vi "BASE_I_O_Manual.vi"(8 "error in (no error)":errorcluster) -> (0 "error out":errorcluster)   [LabVIEW 2017]
doc: "This vi is for manually turn ON and OFF also monitor Output of PLCS. So this is manual screen."
uses:
  Global/PLC_to_Auto.vi
panel:
  in  "Tab Control":enum32{"MANUAL SWITCH", "SCANNER"}(tab)
  in  "Cluster - Thin Border":T1
  in  "Back":bool
  out "Input Signal":T2
  in  "Flush Scaner":bool
  out "SCANNED STRING":string
  in  "Leght of byte to read":bool
  in  "scan":bool
  out "SCANNED COM PORT":refnum<visa-resource-name>
  out "error out 3":errorcluster
  out "error out 4":errorcluster
  # "BARCODE VERIFICATION SYSTEM REPORTS"
  # "Manual Cycle"
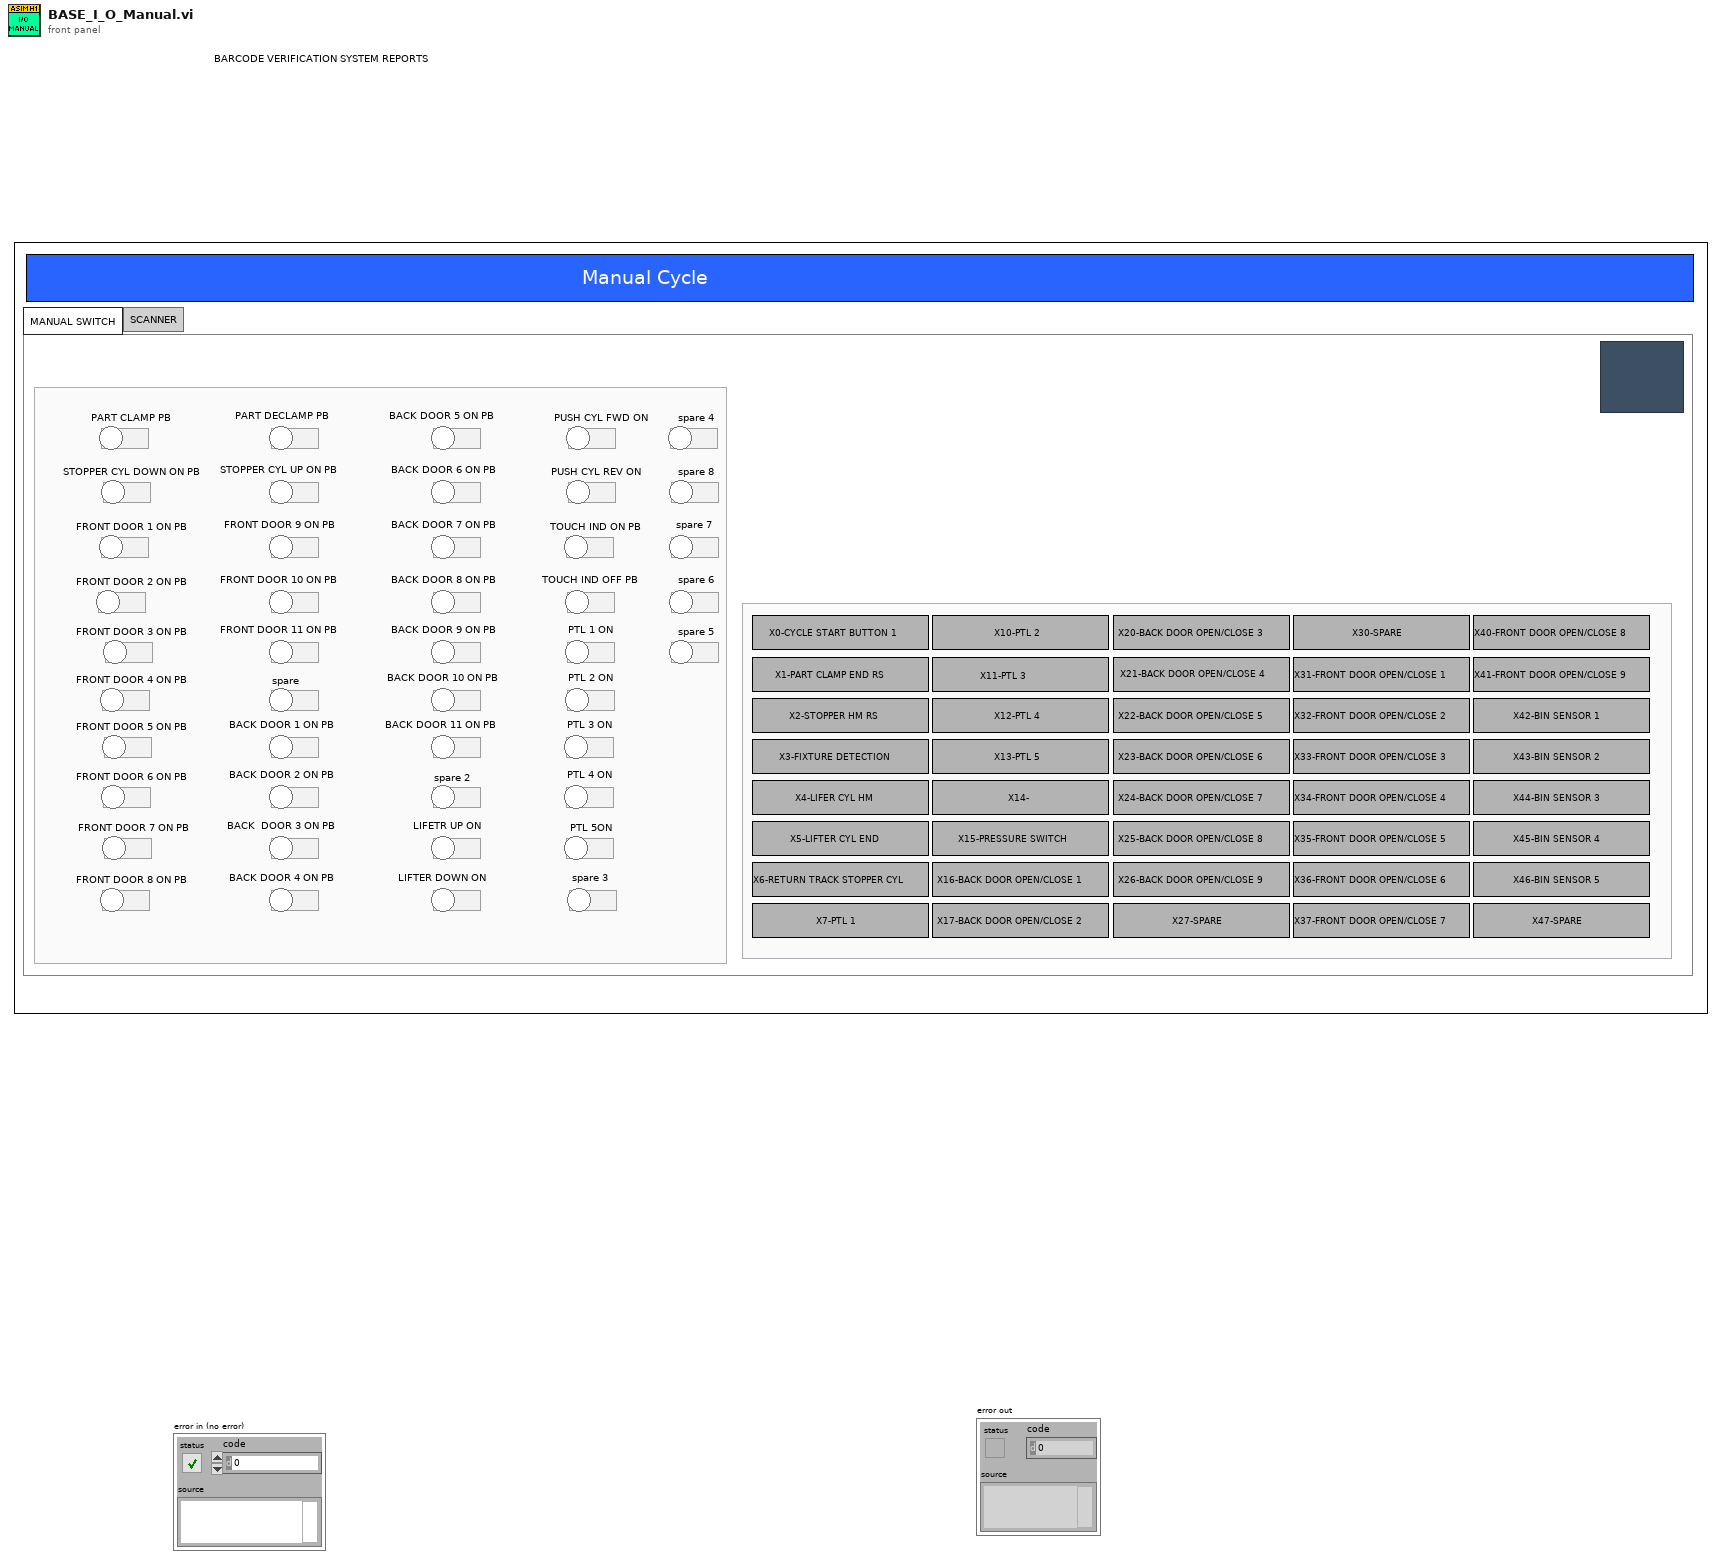
[diagram p1: front panel]
types:
  T1 = cluster{"PART CLAMP PB":bool, "PART DECLAMP PB":bool, "STOPPER CYL DOWN ON PB":bool, "STOPPER CYL UP ON PB":bool, "FRONT DOOR 1 ON PB":bool, "FRONT DOOR 2 ON PB":bool, "FRONT DOOR 3 ON PB":bool, "FRONT DOOR 4 ON PB":bool, "FRONT DOOR 5 ON PB":bool, "FRONT DOOR 6 ON PB":bool, "FRONT DOOR 7 ON PB":bool, "FRONT DOOR 8 ON PB":bool, "FRONT DOOR 9 ON PB":bool, "FRONT DOOR 10 ON PB":bool, "FRONT DOOR 11 ON PB":bool, "spare":bool, "BACK DOOR 1 ON PB":bool, "BACK DOOR 2 ON PB":bool, "BACK  DOOR 3 ON PB":bool, "BACK DOOR 4 ON PB":bool, "BACK DOOR 5 ON PB ":bool, "BACK DOOR 6 ON PB":bool, "BACK DOOR 7 ON PB":bool, "BACK DOOR 8 ON PB":bool, "BACK DOOR 9 ON PB":bool, "BACK DOOR 10 ON PB":bool, "BACK DOOR 11 ON PB\t":bool, "spare 2":bool, "LIFETR UP ON":bool, "LIFTER DOWN ON\t":bool, "PUSH CYL FWD ON\t":bool, "PUSH CYL REV ON":bool, "TOUCH IND ON PB\t":bool, "TOUCH IND OFF PB\t":bool, "PTL 1 ON":bool, "PTL 2 ON\t":bool, "PTL 3 ON":bool, "PTL 4 ON":bool, "PTL 5ON\t":bool, "spare 3":bool, "spare 4":bool, "spare 8":bool, "spare 7":bool, "spare 6":bool, "spare 5":bool}
  T2 = cluster{"CYCLE START TOUCH BUTTON 1":bool, "CYCLE START TOUCH BUTTON 2":bool, "EMG STOP":bool, "RESET PB":bool, "PRESSURE SWITCH":bool, "SAFETY SENSOR":bool, "DOOR 1":bool, "DOOR 2":bool, "SPARE":bool, "SHUTTLE OPEN CHECK SENSOR-X300":bool, "THREAD LOCKER CYL COMPLETE":bool, "PUSHER HM RS":bool, "PUSHER END RS":bool, "UP DOWN CYL  HM RS":bool, "UP DOWN CYL END RS":bool, "PART CLAMP END RS":bool, "X22-DOOR 3":bool, "X23-DOOR 4":bool, "X24-REJECTION SENSOR":bool, "X25-REJECTION FULL SENSOR":bool, "X26-SPARE":bool, "X27-SPARE":bool, "X26-SPARE 2":bool, "X27-SPARE 2":bool, "X26-SPARE 3":bool, "X27-SPARE 3":bool, "X26-SPARE 4":bool, "X27-SPARE 4":bool, "X26-SPARE 5":bool, "X27-SPARE 5":bool, "X26-SPARE 6":bool, "X27-SPARE 6":bool, "X26-SPARE 7":bool, "X27-SPARE 7":bool, "X26-SPARE 8":bool, "X27-SPARE 8":bool, "X26-SPARE 9":bool, "X27-SPARE 9":bool, "X26-SPARE 10":bool, "X27-SPARE 10":bool}
  T3 = cluster{"IP Address":string, "LH Scanner IP Address":string, "RH Scanner IP Address":string}
  T4 = cluster{"[0]":bool, "[1]":bool, "[2]":bool, "[3]":bool, "[4]":bool, "[5]":bool, "[6]":bool, "[7]":bool, "[8]":bool, "[9]":bool, "[10]":bool, "[11]":bool, "[12]":bool, "[13]":bool, "[14]":bool, "[15]":bool, "[16]":bool, "[17]":bool, "[18]":bool, "[19]":bool, "[20]":bool, "[21]":bool, "[22]":bool, "[23]":bool, "[24]":bool, "[25]":bool, "[26]":bool, "[27]":bool, "[28]":bool, "[29]":bool, "[30]":bool, "[31]":bool, "[32]":bool, "[33]":bool, "[34]":bool, "[35]":bool, "[36]":bool, "[37]":bool, "[38]":bool, "[39]":bool}
  T5 = enum32{"invalid app kind", "Development System", "Run Time System", "Student Edition", "Embedded LabVIEW", "Evaluation", "Custom"}
  T6 = enum32{"Invalid", "Standard", "Closed", "Hidden", "Minimized", "Maximized"}
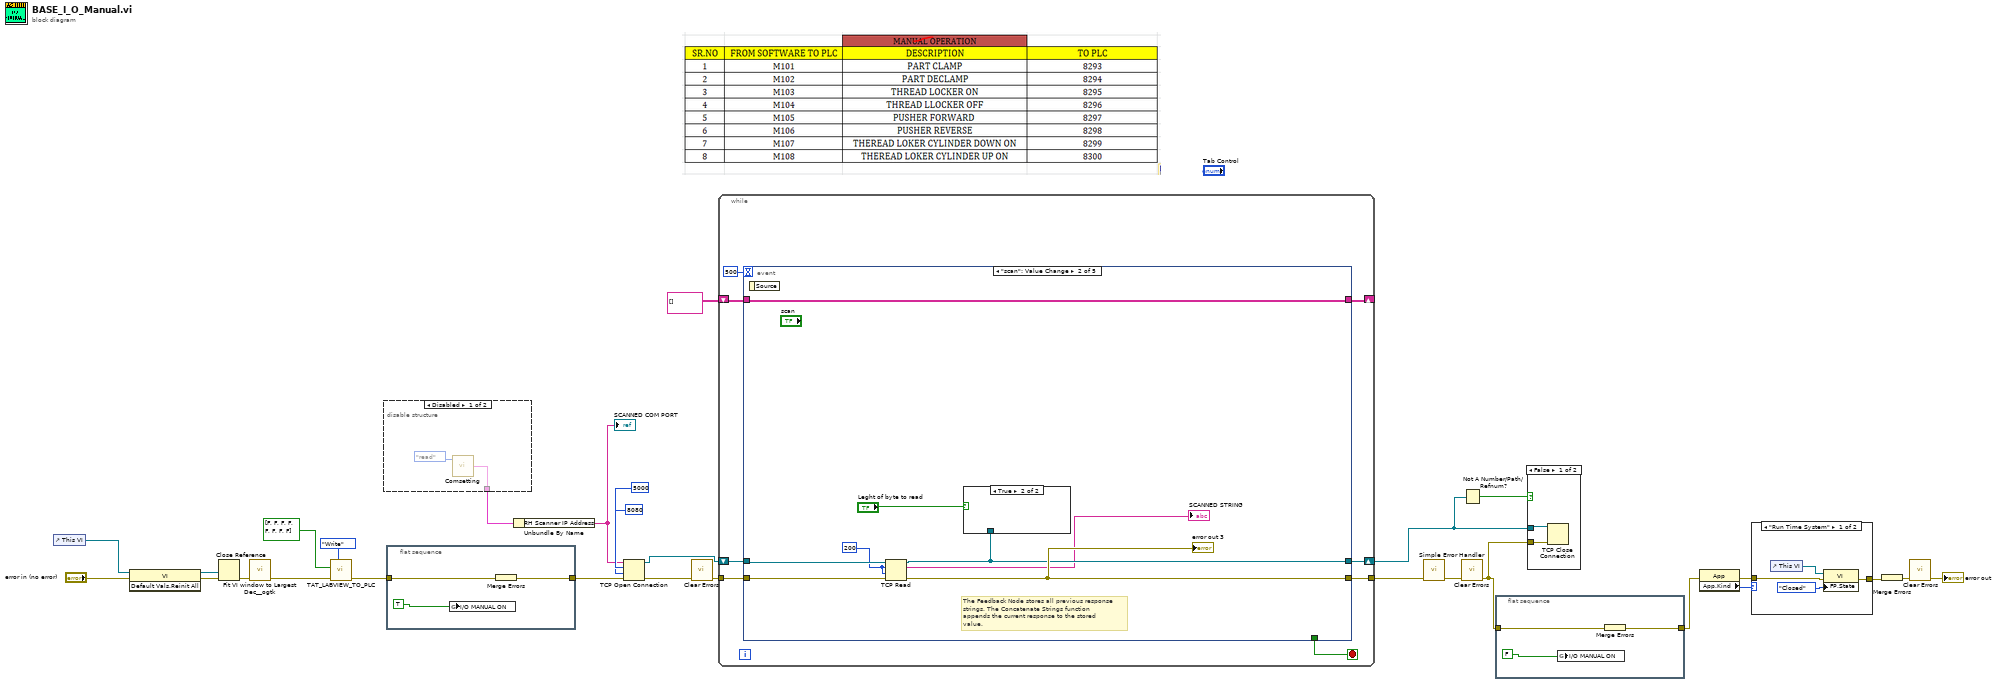
[diagram p0: block diagram]
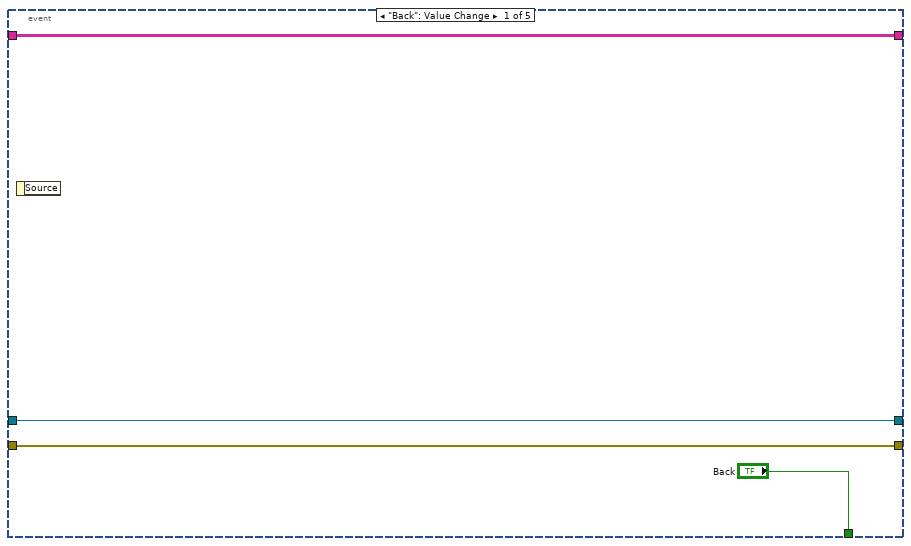
[diagram p5: hidden frame]
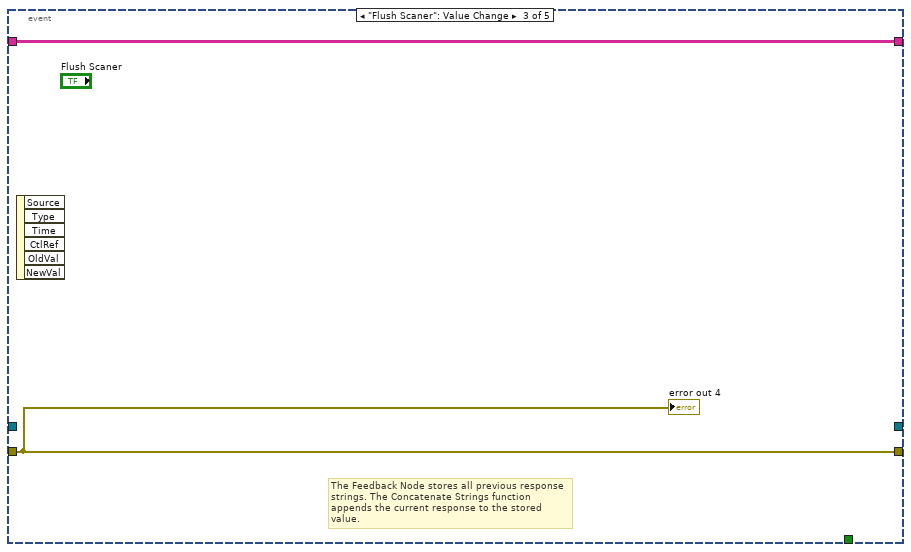
[diagram p7: hidden frame]
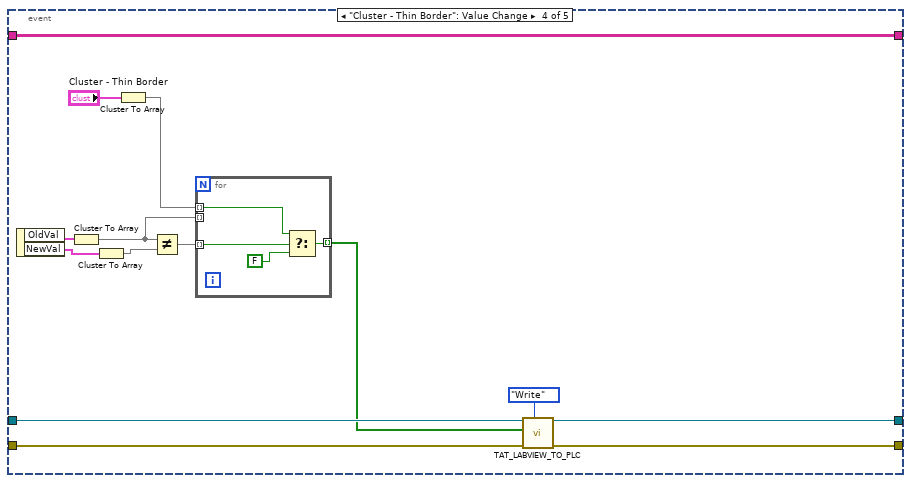
[diagram p8: hidden frame]
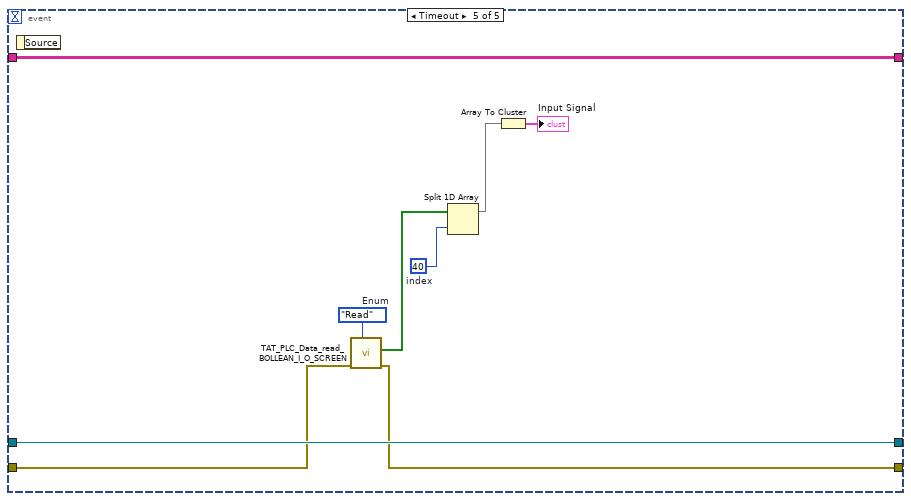
[diagram p9: hidden frame]
diagram:
  n1 = control-ref of="This VI"() -> (w24:refnum<vi>)
  n2 = invoke class="VI" method="Default Vals.Reinit All"(reference=w24, error in="error in (no error)") -> (reference out=w22:refnum<vi>, error out=w21:errorcluster)  [unwired: 1 in, 1 out]
  n3 = Close Reference(reference=w22, error in (no error)=w21) -> (error out=w20:errorcluster)
  n4 = call <userlib>:"Fit VI window to Largest Dec__ogtk.vi"("error in (no error)"=w20) -> ("error out"=w11:errorcluster)  [unwired: 5 in, 1 out]
  n5 = call "TAT_LABVIEW_TO_PLC.vi"("Enum"=enum16{"Read", "Write"}."Write", "error in (no error)"=w11, "Array"=bool[] [FALSE, FALSE, FALSE, FALSE, FALSE, FALSE, FALSE, FALSE]) -> ("error out"=w10:errorcluster)  [unwired: 7 in, 1 out]
  n6 = disable-structure shown="Disabled" {
    disable-tunnel: [w30 _] -> w16
    frame Disabled {
      n7 = call "Comsetting.vi"("Enum"=enum16{"read", "write"}."read") -> ("Cluster Out"=w30:T3)  [unwired: 2 in, 2 out]
    }
    frame Enabled {
    }
  }
  n8 = flat-sequence {
    tunnel: w10 -> [w34]
    tunnel: [w33] -> w15
    frame #0 {
      n9 = global write "PLC_to_Auto.vi" "I/O MANUAL ON"(TRUE) -> ()
      n10 = Merge Errors(w34) -> (w33:errorcluster)
    }
  }
  n11 = Unbundle By Name(w16) -> ("RH Scanner IP Address"=w3:string)
  "SCANNED COM PORT" <- w3
  n12 = TCP Open Connection(address=w3, remote port or service name=u16 8080, timeout ms (60000)=5000, error in (no error)=w15) -> (connection ID=w2:refnum<k5>, error out=w5:errorcluster)  [unwired: 1 in]
  n13 = call <vilib>:"Clear Errors.vi"("error in (no error)"=w5) -> ("error out"=w6:errorcluster)  [unwired: 5 in, 1 out]
  n14 = while {
    tunnel: w6 -> [w42]
    tunnel: [w41] -> w28
    shift-right: [w39] -> _
    shift-left: string[][] [] -> [w38]
    shift-right: [w36] -> w7
    shift-left: w2 -> [w37]
    stop <- w40 stop-if-true
    n15 = event shown="[1] \"scan\": Value Change" {
      selector: _ -> [_ _ _ _ _]
      dyn-events: _ -> [_ _ _ _ _]
      timeout: 500 -> [_ _ _ _ _]
      tunnel: w42 -> [w45 w53 w55 w66 w79]
      tunnel: [w45 w51 w55 w65 w78] -> w41
      tunnel: ["Back" _ _ _ _] -> w40
      tunnel: [w44 w54 w56 w68 w82] -> w39
      tunnel: w38 -> [w44 w54 w56 w68 w82]
      tunnel: w37 -> [w43 w50 _ w69 w81]
      tunnel: [w43 w49 _ w69 w81] -> w36
      event "Back": Value Change {
        n16 = event-data() -> ()  [unwired: 1 in, 1 out]
      }
      event "scan": Value Change {
        w47 = 200 ("bytes to read")
        # "The Feedback Node stores all previous response strings. The Concatenate Strings function appends the current response to the stored value."
        n17 = event-data() -> ()  [unwired: 1 in, 1 out]
        n18 = TCP Read(connection ID=w50, bytes to read=w47, error in (no error)=w53, 9:w47) -> (connection ID out=w49:refnum<k5>, data out=→"SCANNED STRING":string, error out=w51:errorcluster)  [unwired: 1 in]
        "error out 3" <- w51
        n19 = case shown="True" "Leght of byte to read" {
          tunnel: w49 -> [_ _]
          frame False {
          }
          frame True {
          }
        }
      }
      event "Flush Scaner": Value Change {
        # "The Feedback Node stores all previous response strings. The Concatenate Strings function appends the current response to the stored value."
        n20 = event-data() -> ()  [unwired: 1 in, 6 out]
        "error out 4" <- w55
      }
      event "Cluster - Thin Border": Value Change {
        n21 = event-data() -> ("OldVal"=w63:T1, "NewVal"=w62:T1)  [unwired: 1 in]
        n22 = Cluster To Array(cluster=w63) -> (array=w60:bool[])
        n23 = Cluster To Array(cluster=w62) -> (array=w61:bool[])
        n24 = Cluster To Array(cluster="Cluster - Thin Border") -> (array=w58:bool[])
        n25 = Not Equal?(x=w60, y=w61) -> (x != y?=w59:bool[])
        n26 = for {
          tunnel: w58 -> [w72] mode=indexing
          tunnel: w60 -> [_] mode=indexing
          tunnel: w59 -> [w73] mode=indexing
          tunnel: [w71] -> w57 mode=indexing
          n27 = Select(t=w72, s=w73, f=FALSE) -> (s? t:f=w71:bool)
        }
        n28 = call "TAT_LABVIEW_TO_PLC.vi"("Enum"=enum16{"Read", "Write"}."Write", "error in (no error)"=w66, "Array"=w57) -> ("error out"=w65:errorcluster)  [unwired: 7 in, 1 out]
      }
      event Timeout {
        w75 = 40  # index
        w80 = enum16{"Read", "Write"}."Read"  # Enum
        n29 = event-data() -> ()  [unwired: 1 in, 1 out]
        n30 = call "TAT_PLC_Data_read_BOLLEAN_I_O_SCREEN.vi"("Enum"=w80, "error in (no error)"=w79) -> ("error out"=w78:errorcluster, "Array 2"=w76:bool[])  [unwired: 8 in]
        n31 = Split 1D Array(array=w76, index=w75) -> (first subarray=w74:bool[])  [unwired: 1 out]
        n32 = Array To Cluster(array=w74) -> (cluster=→"Input Signal":T4)
      }
    }
  }
  n33 = call <vilib>:"Simple Error Handler.vi"("error in (no error)"=w28) -> ("error out"=w19:errorcluster)  [unwired: 4 in, 4 out]
  n34 = call <vilib>:"Clear Errors.vi"("error in (no error)"=w19) -> ("error out"=w14:errorcluster)  [unwired: 5 in, 1 out]
  n35 = Not A Number/Path/Refnum?(number/path/refnum=w7) -> (NaN/Path/Refnum?=w8:bool)
  n36 = flat-sequence {
    tunnel: w14 -> [w85]
    tunnel: [w84] -> w13
    frame #0 {
      n37 = global write "PLC_to_Auto.vi" "I/O MANUAL ON"(FALSE) -> ()
      n38 = Merge Errors(w85) -> (w84:errorcluster)
    }
  }
  n39 = case shown="False" w8 {
    tunnel: w7 -> [w86 _]
    tunnel: w14 -> [w87 _]
    frame False {
      n40 = TCP Close Connection(connection ID=w86, error in (no error)=w87) -> ()  [unwired: 1 in, 2 out]
    }
    frame True {
    }
  }
  n41 = property class="App"(error in=w13) -> (error out=w17:errorcluster, "App.Kind"=w18:T5)  [unwired: 1 in, 1 out]
  n42 = case shown="\"Run Time System\"" w18 {
    tunnel: w17 -> [w89 w92]
    tunnel: [w88 w92] -> w26
    frame "Run Time System" {
      n43 = control-ref of="This VI"() -> (w91:refnum<vi>)
      n44 = property class="VI"(reference=w91, error in=w89, "FP.State"=T6."Closed" ("Front Panel Window:State")) -> (error out=w88:errorcluster)  [unwired: 1 out]
    }
    frame "Development System", Default {
    }
  }
  n45 = Merge Errors(w26) -> (w27:errorcluster)
  n46 = call <vilib>:"Clear Errors.vi"("error in (no error)"=w27) -> ("error out"=→"error out":errorcluster)  [unwired: 5 in, 1 out]
